vi "Parse Low-Side Driver + Wheel Overcurrents.vi"(11 "stream in":u8[](array[numeric])) -> (0 "Low-Side Driver + Wheel Overcurrent":T1, 3 "stream out":u8[](array[numeric]))   [LabVIEW 2013]
doc: "Read the state of low-side driver and wheel overcurrents from a UART data stream."
uses:
  Low-Side Driver + Wheel Overcurrent.ctl
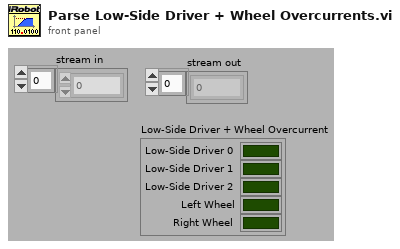
[diagram p1: front panel]
types:
  T1 = typedef "Low-Side Driver + Wheel Overcurrent.ctl" = cluster{"Low-Side Driver 0":bool, "Low-Side Driver 1":bool, "Low-Side Driver 2":bool, "Left Wheel":bool, "Right Wheel":bool}
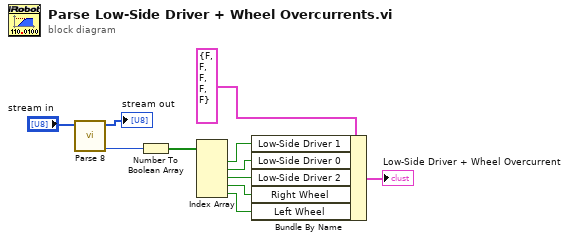
[diagram p0: block diagram]
diagram:
  n1 = call "Parse 8.vi"("stream in"="stream in") -> ("value"=w1:u8, "stream out"=→"stream out":u8[])  [unwired: 9 out]
  n2 = Number To Boolean Array(number=w1) -> (Boolean array=w11:bool[])
  n3 = Index Array(array=w11) -> (element #1=w10:bool, element #2=w9:bool, element #3=w8:bool, element #4=w7:bool, element #5=w6:bool)  [unwired: 5 in]
  n4 = Bundle By Name(cluster=T1 {"Low-Side Driver 0"=FALSE, "Low-Side Driver 1"=FALSE, "Low-Side Driver 2"=FALSE, "Left Wheel"=FALSE, "Right Wheel"=FALSE} ("Low-Side Driver + Wheel Overcurrent"), "Low-Side Driver 1"=w10, "Low-Side Driver 0"=w9, "Low-Side Driver 2"=w8, "Right Wheel"=w7, "Left Wheel"=w6) -> (→"Low-Side Driver + Wheel Overcurrent":T1)
